vi "get Phasor Config Labview.vi"(6 "phasorIndex":i32, 7 "pmuIndex":i32, 9 "pseudoPdcId":i32, 10 "name":string, 11 "phasorCfg":T1) -> (1 "function return":i32, 2 "name out":string, 3 "phasorCfg out":T1)   [LabVIEW 2013, in "C37118-DLL.lvlib" / "StrongridDLL.lvlib"]
doc: "STRONGRIDIEEEC37118DLL_API int __cdecl getPhasorConfigLabview(noArraysPhasorConfig *phasorCfg, char* name, int32_t pseudoPdcId, int32_t pmuIndex, int32_t phasorIndex);"
uses:
  StrongridDLL.lvlib
  builds/StrongridDLL/StrongridDLL.dll
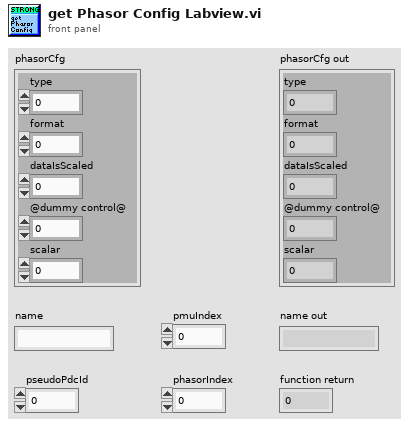
[diagram p1: front panel]
types:
  T1 = cluster{"type":u8, "format":u8, "dataIsScaled":u8, "@dummy control@":i8, "scalar":sgl}
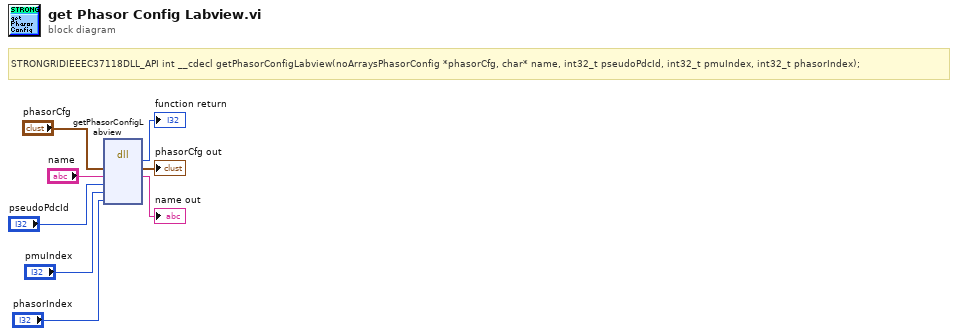
[diagram p0: block diagram]
diagram:
  # "STRONGRIDIEEEC37118DLL_API int __cdecl getPhasorConfigLabview(noArraysPhasorConfig *phasorCfg, char* name, int32_t pseudoPdcId, int32_t pmuIndex, int32_t phasorIndex);"
  n1 = dll-call lib="C:/dev/OSS/S3DK/builds/StrongridDLL/StrongridDLL.*" fn="getPhasorConfigLabview"("phasorCfg"="phasorCfg", "name"="name", "pseudoPdcId"="pseudoPdcId", "pmuIndex"="pmuIndex", "phasorIndex"="phasorIndex") -> (→"function return":i32, "phasorCfg"=→"phasorCfg out":T1, "name"=→"name out":string)  [unwired: 6 in, 2 out]
